vi "_old_Load_HW_globals.vi"(0 "HW settings path":path=path "C:/Experiment/Data Acquisition/Hardware Control/procedures/23Apr09_Example", 1 "Load pre 5.6 Globals?":bool, 2 "Pre 4.1 HWGlobals?":bool, 5 "error in":errorcluster) -> (6 "Loaded Procedure Data":T1={"User defined functions"="\n-- -------------------------------------------------------------------------------------------\n-- The following functions are part of the \"standard load\" of functions and should not be messed with\n-- They are here for reference only.\n-- Please add any user functions above this comment\n-- -------------------------------------------------------------------------------------------\n\n-- Creates a linear ramp from A to B\nfunction LineRamp(f, Initial, Final)\n    return (1-f)*Initial + f*Final;\nend\n\n-- Creates an exponential ramp from A to B\nfunction ExpRamp(t, a, b, tau)\n   return (b - a*exp(tMax / tau) + (a-b)*exp(t/tau))/ ( 1 - exp(tMax / tau) );\nend\n\n-- Creates a sinewave\nfunction SinRamp(t,Offset,A,Freq, Phase)\n    return Offset + A * sin(2*pi*Freq*t + Phase)\nend\n\n-- Creates a blackman pulse\nfunction Blackman(f, Offset, A)\n    return Offset +  A*sqrt(0.5*cos(3.1415*(2*f-1))+0.08*cos(2*pi*(2*f-1))+0.42);\nend\n\n-- Creates a half-gauss ramp\nfunction HalfGaussRamp(t, a, b, Width)\n    local y;\n    y = exp(-(tMax^2)/Width^2);\n    y = (a -  b*y)/(1-y)  +  ((b-a)/(1-y))*exp(-((t-tMax)^2)/Width^2);\n    return y;\nend\n\n-- Creates an \"O'Hara\" ramp from A to B, for dipole evaporation\nfunction EvapRamp(t, a, b, tau)\n   local y;\n  y = log(a/b) / log(1+tMax/tau);\n  y = a * (1+t/tau)^(-y);\n  return y;\nend\n", "Master AO Channels"=[], "Novatech Devices"=[], "DDS Devices"=[]}, 7 "Profile Name":string="IBS_PICameraTest_29Sep04", 8 "error out":errorcluster)   [LabVIEW 2013]
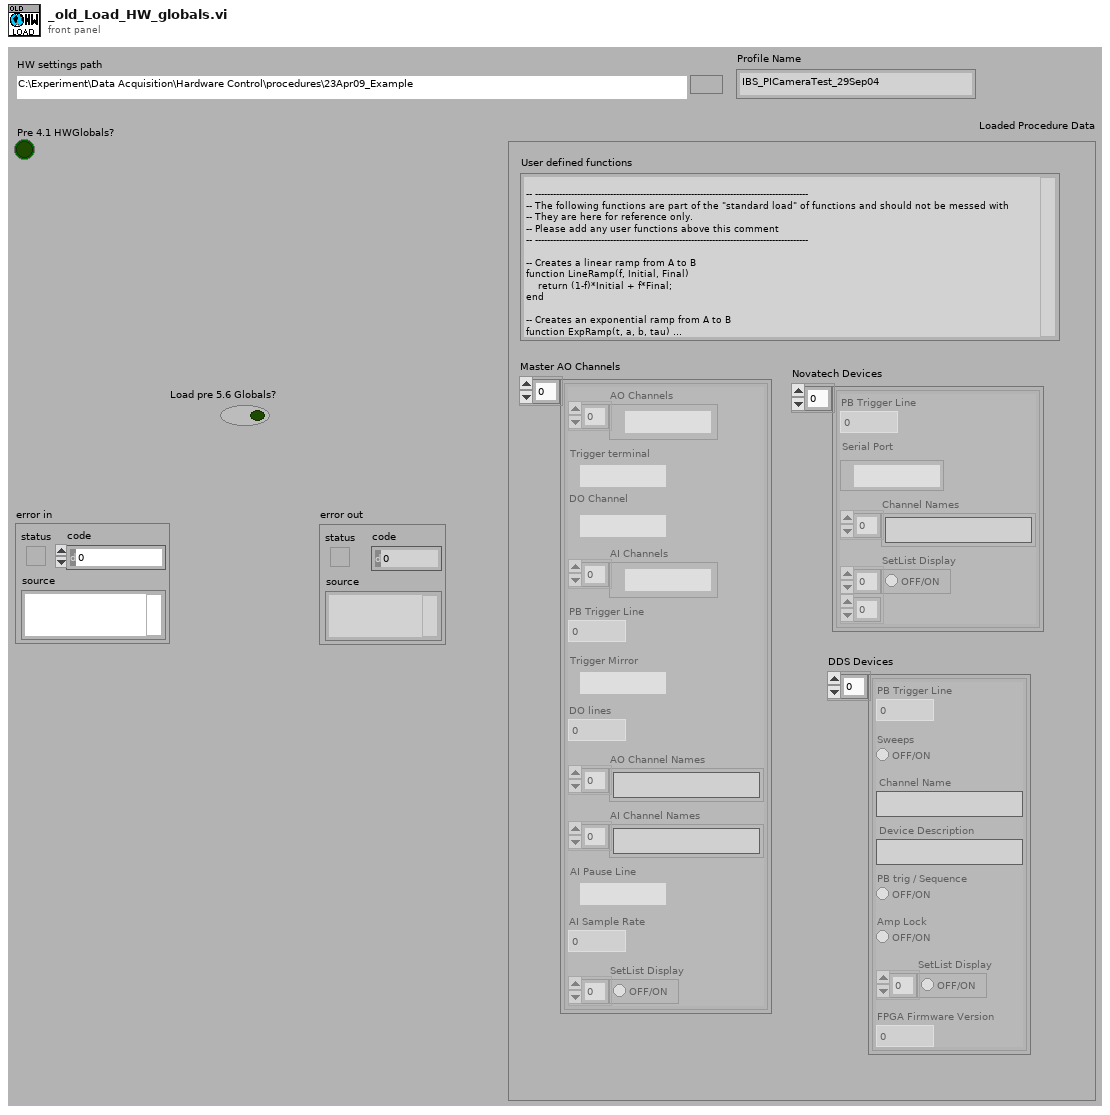
[diagram p1: front panel]
types:
  T1 = cluster{"User defined functions":string, "Master AO Channels":cluster{"AO Channels":refnum<k21>[], "Trigger terminal":tag, "DO Channel":refnum<k21>, "AI Channels":refnum<k21>[], "PB Trigger Line":u16, "Trigger Mirror":tag, "DO lines":i32, "AO Channel Names":string[], "AI Channel Names":string[], "AI Pause Line":tag, "AI Sample Rate":dbl, "SetList Display":bool[]}[], "Novatech Devices":cluster{"PB Trigger Line":u16, "Serial Port":refnum<visa-resource-name>, "Channel Names":string[], "SetList Display":bool[][]}[], "DDS Devices":cluster{"PB Trigger Line":u16, "Sweeps":bool, "Channel Name":string, "Device Description":string, "PB trig / Sequence":bool, "Amp Lock":bool, "SetList Display":bool[], "FPGA Firmware Version":dbl}[]}
  T2 = cluster{"PB Trigger Line":u16, "Serial Port":refnum<visa-resource-name>, "Channel Names":string[], "SetList Display":bool[][]}
  T3 = cluster{"AO Channels":refnum<k21>[], "Trigger terminal":tag, "DO Channel":refnum<k21>, "AI Channels":refnum<k21>[], "PB Trigger Line":u16, "Trigger Mirror":tag, "DO lines":i32, "AO Channel Names":string[], "AI Channel Names":string[], "AI Pause Line":tag, "AI Sample Rate":dbl, "SetList Display":bool[]}
  T4 = cluster{"PB Trigger Line":u16, "Sweeps":bool, "Channel Name":string, "Device Description":string, "PB trig / Sequence":bool, "Amp Lock":bool, "SetList Display":bool[], "FPGA Firmware Version":dbl}
  T5 = cluster{"PB Trigger Line":u16, "Sweeps":bool, "Channel Name":string, "Device Description":string, "PB trig / Sequence":bool, "Amp Lock":bool, "SetList Display":bool[], "FPGA Firmware Version":dbl}[]
  T6 = cluster{"PB Trigger Line":u16, "Sweeps":bool, "Channel Name":string, "Device Description":string, "PB trig / Sequence":bool, "Amp Lock":bool, "SetList Display":bool[]}
  T7 = cluster{"PB Trigger Line":u16, "Sweeps":bool, "Channel Name":string, "Device Description":string, "PB trig / Sequence":bool, "Amp Lock":bool, "SetList Display":bool[]}[]
  T8 = cluster{"PB Trigger Line":u16, "Serial Port":refnum<visa-resource-name>, "Channel Names":string[]}
  T9 = cluster{"PB Trigger Line":u16, "Serial Port":refnum<visa-resource-name>, "Channel Names":string[], "SetList Display":bool[][]}[]
  T10 = cluster{"AO Channels":refnum<k21>[], "Trigger terminal":tag, "DO Channel":refnum<k21>, "AI Channels":refnum<k21>[], "PB Trigger Line":u16, "Trigger Mirror":tag, "DO lines":i32, "AO Channel Names":string[], "AI Channel Names":string[], "AI Pause Line":tag, "AI Sample Rate":dbl}
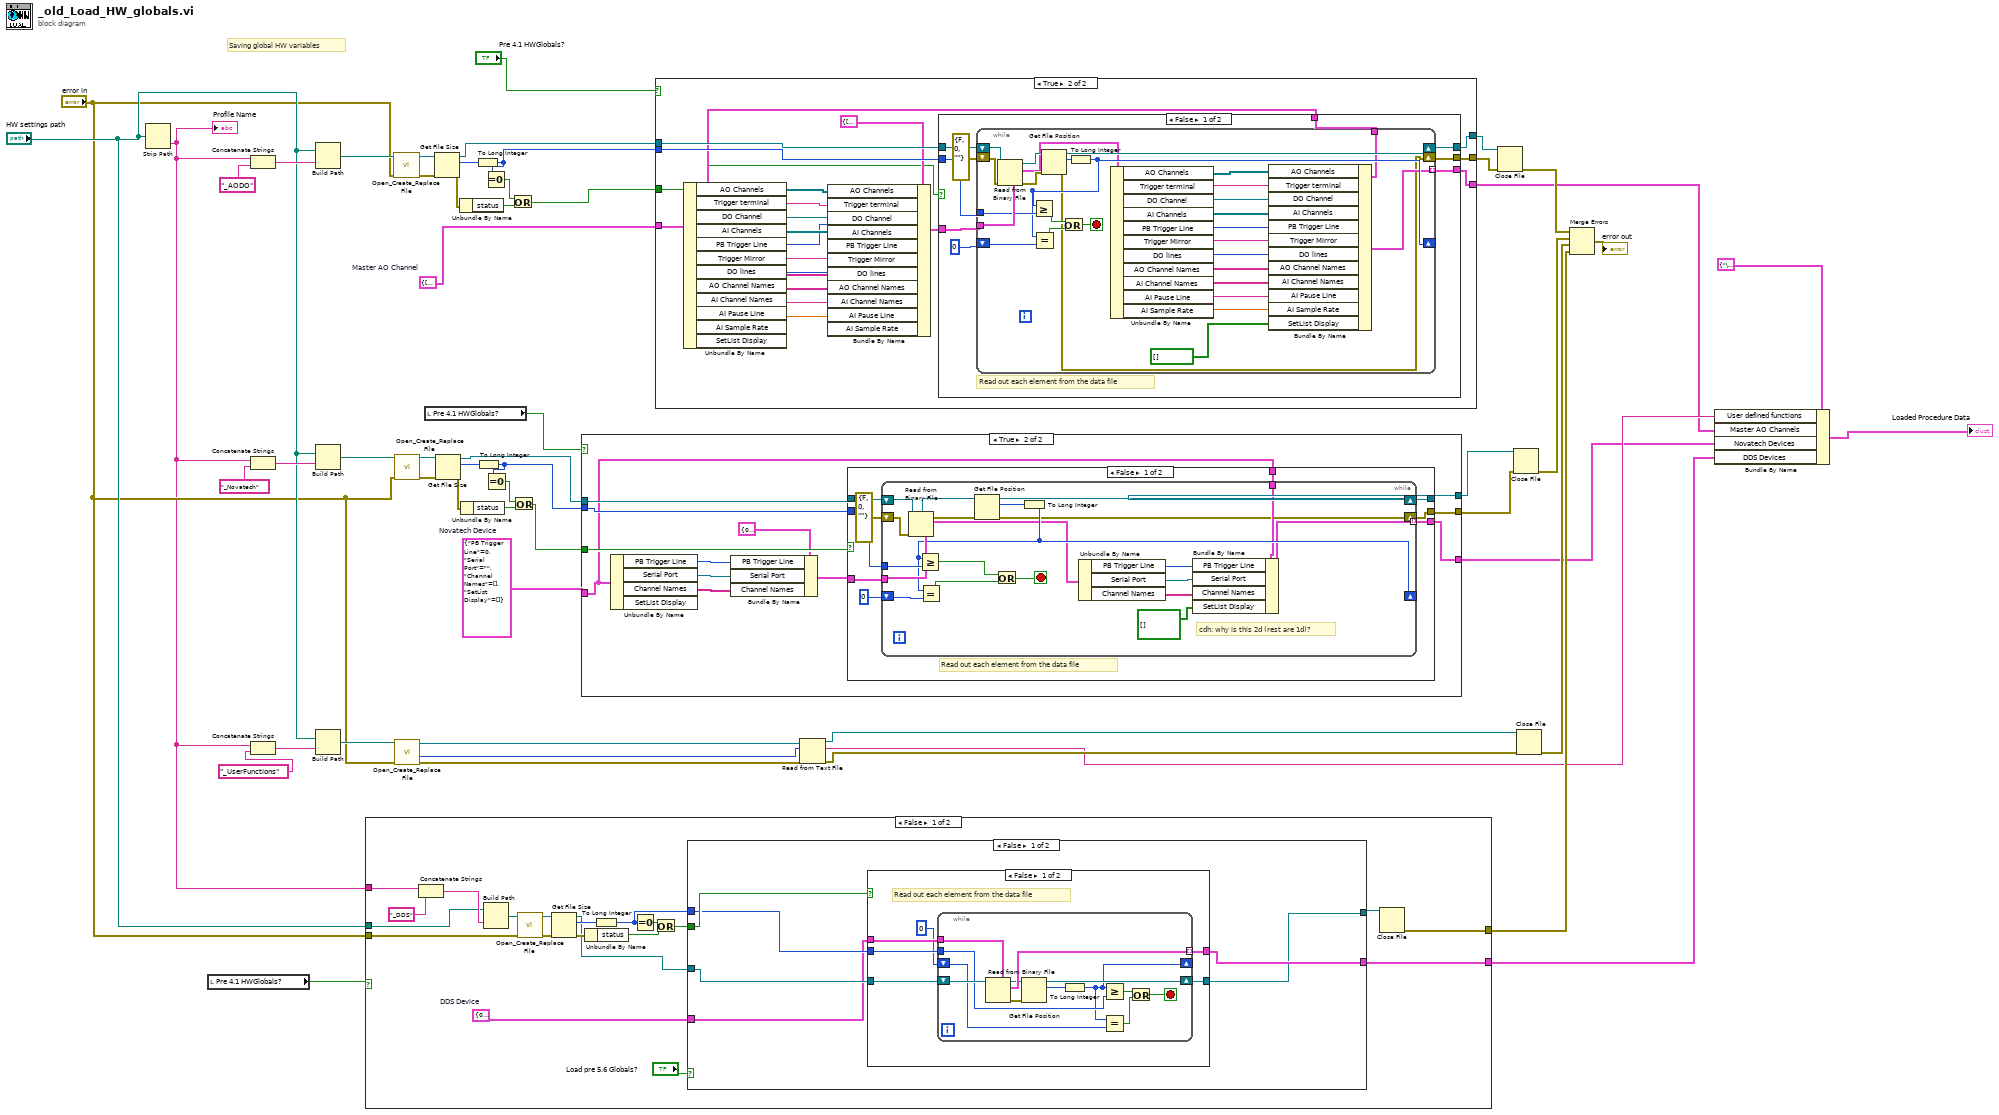
[diagram p0: block diagram]
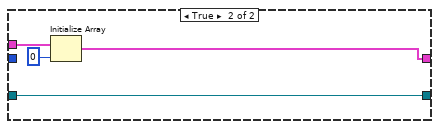
[diagram p2: hidden frame]
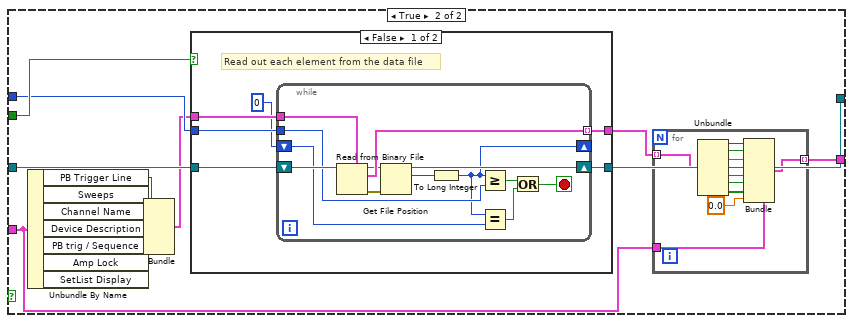
[diagram p3: hidden frame]
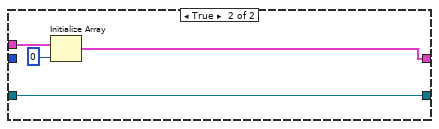
[diagram p4: hidden frame]
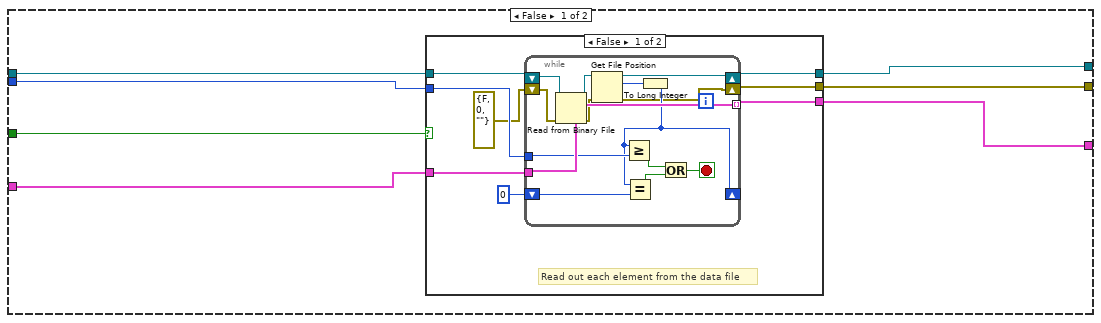
[diagram p6: hidden frame]
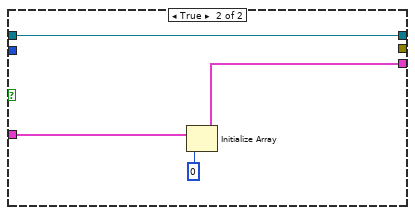
[diagram p7: hidden frame]
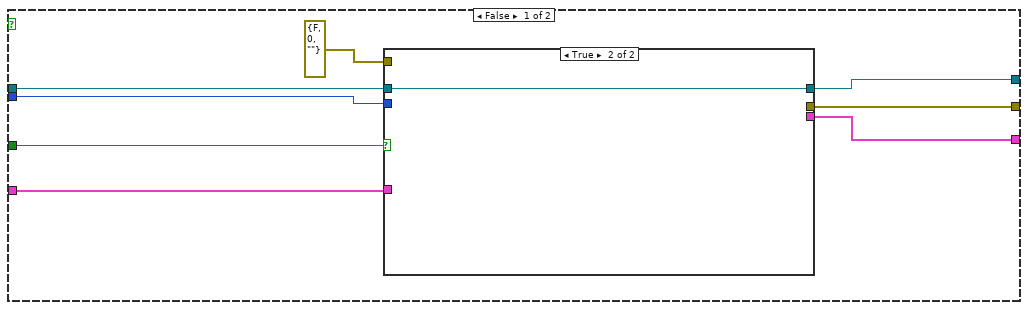
[diagram p9: hidden frame]
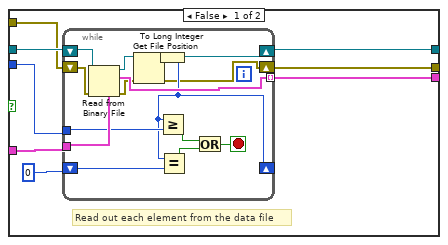
[diagram p10: hidden frame]
diagram:
  w5 = T2 {"PB Trigger Line"=0, "Serial Port"="", "Channel Names"=[], "SetList Display"=[]}  # Novatech Device
  w16 = T3 {"AO Channels"=[], "Trigger terminal"="", "DO Channel"="", "AI Channels"=[], "PB Trigger Line"=0, "Trigger Mirror"="", "DO lines"=0, "AO Channel Names"=[], "AI Channel Names"=[], "AI Pause Line"="", "AI Sample Rate"=0.0, "SetList Display"=[]}  # Master AO Channel
  # "Saving global HW variables"
  n1 = Strip Path(path="HW settings path") -> (name=w22:string)  [unwired: 1 out]
  "Profile Name" <- w22
  n2 = local read "Pre 4.1 HWGlobals?"() -> (w1:bool)
  n3 = Concatenate Strings(w22, "_AODO") -> (w54:string)
  n4 = Concatenate Strings(w22, "_Novatech") -> (w52:string)
  n5 = Concatenate Strings(w22, "_UserFunctions") -> (w33:string)
  n6 = Build Path(base path="HW settings path", name or relative path=w54) -> (appended path=w44:path)
  n7 = Build Path(base path="HW settings path", name or relative path=w52) -> (appended path=w37:path)
  n8 = Build Path(base path="HW settings path", name or relative path=w33) -> (appended path=w32:path)
  n9 = case shown="False" w1 {
    tunnel: "HW settings path" -> [w62 _]
    tunnel: "error in" -> [w61 _]
    tunnel: [w60 _] -> w23
    tunnel: w22 -> [w59 _]
    tunnel: [w56 _] -> w19
    frame False {
      w57 = T4 {"PB Trigger Line"=0, "Sweeps"=FALSE, "Channel Name"="", "Device Description"="", "PB trig / Sequence"=FALSE, "Amp Lock"=FALSE, "SetList Display"=[], "FPGA Firmware Version"=0.0}  # DDS Device
      n10 = Concatenate Strings(w59, "_DDS") -> (w64:string)
      n11 = Build Path(base path=w62, name or relative path=w64) -> (appended path=w75:path)
      n12 = call <vilib>:"Open_Create_Replace File.vi"("error in (no error)"=w61, "file path"=w75) -> ("error out"=w73:errorcluster, "refnum"=w66:refnum<file>)  [unwired: 4 in, 4 out]
      n13 = Get File Size(file=w66, error in=w73) -> (refnum out=w67:refnum<file>, size (in bytes)=w69:i64, 0:w74:errorcluster)
      n14 = Unbundle By Name(w74) -> ("status"=w72:bool)
      n15 = To Long Integer(number=w69) -> (32bit integer=w68:i32)
      n16 = Equal To 0?(x=w68) -> (x = 0?=w71:bool)
      n17 = Or(x=w71, y=w72) -> (x .or. y?=w70:bool)
      n18 = case shown="False" "Load pre 5.6 Globals?" {
        tunnel: w70 -> [w80 w119]
        tunnel: w68 -> [w79 w118]
        tunnel: w67 -> [w81 w117]
        tunnel: [w76 w116] -> w65
        tunnel: w57 -> [w78 w106]
        tunnel: [w77 w105] -> w56
        frame False {
          n19 = case shown="False" w80 {
            tunnel: [w87 w104] -> w76
            tunnel: w78 -> [w86 w102]
            tunnel: w81 -> [w85 w104]
            tunnel: [w84 w103] -> w77
            tunnel: w79 -> [w83 _]
            frame False {
              # "Read out each element from the data file"
              n20 = while {
                tunnel: [w98] -> w84 mode=indexing
                tunnel: w86 -> [w97]
                shift-right: [w99] -> w87
                shift-left: w85 -> [w100]
                tunnel: w83 -> [w96]
                shift-right: [w95] -> _
                shift-left: 0 -> [w94]
                stop <- w91 stop-if-true
                n21 = Read from Binary File(5:w97, 11:w100) -> (0:w89:errorcluster, 2:w98:T4, 3:w90:refnum<file>)  [unwired: 1 in, 4 out]
                n22 = Get File Position(4:w89, 7:w90) -> (2:w88:i64, 3:w99:refnum<file>)  [unwired: 1 out]
                n23 = To Long Integer(number=w88) -> (32bit integer=w95:i32)
                n24 = Greater Or Equal?(x=w95, y=w96) -> (x >= y?=w92:bool)
                n25 = Equal?(x=w95, y=w94) -> (x = y?=w93:bool)
                n26 = Or(x=w92, y=w93) -> (x .or. y?=w91:bool)
              }
            }
            frame True {
              n27 = Initialize Array(w102, 0) -> (w103:T5)
            }
          }
        }
        frame True {
          n28 = Unbundle By Name(w106) -> ("PB Trigger Line"=w109:u16, "Sweeps"=w115:bool, "Channel Name"=w114:string, "Device Description"=w113:string, "PB trig / Sequence"=w112:bool, "Amp Lock"=w111:bool, "SetList Display"=w110:bool[])
          n29 = Bundle("PB Trigger Line"=w109, "Sweeps"=w115, "Channel Name"=w114, "Device Description"=w113, "PB trig / Sequence"=w112, "Amp Lock"=w111, "SetList Display"=w110) -> (w108:T6)  [unwired: 1 in]
          n30 = case shown="False" w119 {
            tunnel: [w136 w153] -> w116
            tunnel: w108 -> [w135 w151]
            tunnel: w117 -> [w134 w153]
            tunnel: [w133 w152] -> w107
            tunnel: w118 -> [w132 _]
            frame False {
              # "Read out each element from the data file"
              n31 = while {
                tunnel: [w147] -> w133 mode=indexing
                tunnel: w135 -> [w146]
                shift-right: [w148] -> w136
                shift-left: w134 -> [w149]
                tunnel: w132 -> [w145]
                shift-right: [w144] -> _
                shift-left: 0 -> [w143]
                stop <- w140 stop-if-true
                n32 = Read from Binary File(5:w146, 11:w149) -> (0:w138:errorcluster, 2:w147:T6, 3:w139:refnum<file>)  [unwired: 1 in, 4 out]
                n33 = Get File Position(4:w138, 7:w139) -> (2:w137:i64, 3:w148:refnum<file>)  [unwired: 1 out]
                n34 = To Long Integer(number=w137) -> (32bit integer=w144:i32)
                n35 = Greater Or Equal?(x=w144, y=w145) -> (x >= y?=w141:bool)
                n36 = Equal?(x=w144, y=w143) -> (x = y?=w142:bool)
                n37 = Or(x=w141, y=w142) -> (x .or. y?=w140:bool)
              }
            }
            frame True {
              n38 = Initialize Array(w151, 0) -> (w152:T7)
            }
          }
          n39 = for {
            tunnel: w107 -> [w130] mode=indexing
            tunnel: w106 -> [w129]
            tunnel: [w120] -> w105 mode=indexing
            n40 = Unbundle(w130) -> ("PB Trigger Line"=w128:u16, "Sweeps"=w127:bool, "Channel Name"=w126:string, "Device Description"=w125:string, "PB trig / Sequence"=w124:bool, "Amp Lock"=w123:bool, "SetList Display"=w122:bool[])
            n41 = Bundle(cluster=w129, "PB Trigger Line"=w128, "Sweeps"=w127, "Channel Name"=w126, "Device Description"=w125, "PB trig / Sequence"=w124, "Amp Lock"=w123, "SetList Display"=w122, "FPGA Firmware Version"=0.0) -> (w120:T4)
          }
        }
      }
      n42 = Close File(refnum=w65) -> (error out=w60:errorcluster)  [unwired: 1 in, 1 out]
    }
    frame True {
    }
  }
  n43 = call <vilib>:"Open_Create_Replace File.vi"("error in (no error)"="error in", "file path"=w44) -> ("error out"=w46:errorcluster, "refnum"=w50:refnum<file>)  [unwired: 4 in, 4 out]
  n44 = call <vilib>:"Open_Create_Replace File.vi"("error in (no error)"="error in", "file path"=w37) -> ("error out"=w39:errorcluster, "refnum"=w43:refnum<file>)  [unwired: 4 in, 4 out]
  n45 = call <vilib>:"Open_Create_Replace File.vi"("error in (no error)"="error in", "file path"=w32) -> ("error out"=w28:errorcluster, "file size (bytes)"=w29:i32, "refnum"=w30:refnum<file>)  [unwired: 4 in, 3 out]
  n46 = local read "Pre 4.1 HWGlobals?"() -> (w6:bool)
  n47 = Get File Size(file=w50, error in=w46) -> (refnum out=w14:refnum<file>, size (in bytes)=w49:i64, 0:w45:errorcluster)
  n48 = Get File Size(file=w43, error in=w39) -> (refnum out=w7:refnum<file>, size (in bytes)=w42:i64, 0:w38:errorcluster)
  n49 = Unbundle By Name(w45) -> ("status"=w47:bool)
  n50 = Unbundle By Name(w38) -> ("status"=w40:bool)
  n51 = To Long Integer(number=w49) -> (32bit integer=w15:i32)
  n52 = To Long Integer(number=w42) -> (32bit integer=w8:i32)
  n53 = Equal To 0?(x=w15) -> (x = 0?=w48:bool)
  n54 = Equal To 0?(x=w8) -> (x = 0?=w41:bool)
  n55 = Or(x=w48, y=w47) -> (x .or. y?=w17:bool)
  n56 = Or(x=w41, y=w40) -> (x .or. y?=w9:bool)
  n57 = case shown="True" w6 {
    tunnel: [w160 w194] -> w2
    tunnel: w7 -> [w159 w195]
    tunnel: w8 -> [w158 w196]
    tunnel: w9 -> [w157 w193]
    tunnel: w5 -> [w156 w190]
    tunnel: [w155 w189] -> w4
    tunnel: [w154 w188] -> w3
    frame False {
      n58 = case shown="False" w157 {
        tunnel: [w168 w187] -> w160
        tunnel: w156 -> [w167 w185]
        tunnel: w159 -> [w166 w187]
        tunnel: [w165 w186] -> w155
        tunnel: w158 -> [w164 _]
        tunnel: [w162 _] -> w154
        frame False {
          # "Read out each element from the data file"
          n59 = while {
            tunnel: [w181] -> w165 mode=indexing
            tunnel: w167 -> [w180]
            shift-right: [w182] -> w168
            shift-left: w166 -> [w183]
            tunnel: w164 -> [w179]
            shift-right: [w178] -> _
            shift-left: 0 -> [w177]
            shift-right: [w170] -> w162
            shift-left: errorcluster {"status"=FALSE, "code"=0, "source"=""} ("error out") -> [w169]
            stop <- w174 stop-if-true
            n60 = Read from Binary File(5:w180, 8:w169, 11:w183) -> (0:w172:errorcluster, 2:w181:T2, 3:w173:refnum<file>)  [unwired: 4 out]
            n61 = Get File Position(4:w172, 7:w173) -> (0:w170:errorcluster, 2:w171:i64, 3:w182:refnum<file>)
            n62 = To Long Integer(number=w171) -> (32bit integer=w178:i32)
            n63 = Greater Or Equal?(x=w178, y=w179) -> (x >= y?=w175:bool)
            n64 = Equal?(x=w178, y=w177) -> (x = y?=w176:bool)
            n65 = Or(x=w175, y=w176) -> (x .or. y?=w174:bool)
          }
        }
        frame True {
          n66 = Initialize Array(w185, 0) -> (w186:T9)
        }
      }
    }
    frame True {
      n67 = Unbundle By Name(w190) -> ("PB Trigger Line"=w199:u16, "Serial Port"=w198:refnum<visa-resource-name>, "Channel Names"=w197:string[])  [unwired: 1 out]
      n68 = Bundle By Name(cluster=T8 {"PB Trigger Line"=0, "Serial Port"="", "Channel Names"=[]} ("output cluster"), "PB Trigger Line"=w199, "Serial Port"=w198, "Channel Names"=w197) -> (w191:T8)
      n69 = case shown="False" w193 {
        tunnel: [w208 w230] -> w194
        tunnel: w191 -> [w207 _]
        tunnel: w195 -> [w206 w230]
        tunnel: [w205 _] -> w189
        tunnel: w196 -> [w204 _]
        tunnel: w190 -> [w202 _]
        tunnel: [w201 _] -> w188
        frame False {
          # "Read out each element from the data file"
          n70 = while {
            tunnel: [w211] -> w205 mode=indexing
            tunnel: w207 -> [w227]
            shift-right: [w228] -> w208
            shift-left: w206 -> [w229]
            tunnel: w204 -> [w226]
            shift-right: [w225] -> _
            shift-left: 0 -> [w224]
            tunnel: w202 -> [w213]
            shift-right: [w210] -> w201
            shift-left: errorcluster {"status"=FALSE, "code"=0, "source"=""} ("error out") -> [w209]
            stop <- w221 stop-if-true
            # "cdh: why is this 2d (rest are 1d)?"
            n71 = Read from Binary File(5:w227, 8:w209, 11:w229) -> (0:w219:errorcluster, 2:w217:T8, 3:w220:refnum<file>)  [unwired: 4 out]
            n72 = Get File Position(4:w219, 7:w220) -> (0:w210:errorcluster, 2:w218:i64, 3:w228:refnum<file>)
            n73 = To Long Integer(number=w218) -> (32bit integer=w225:i32)
            n74 = Greater Or Equal?(x=w225, y=w226) -> (x >= y?=w222:bool)
            n75 = Equal?(x=w225, y=w224) -> (x = y?=w223:bool)
            n76 = Or(x=w222, y=w223) -> (x .or. y?=w221:bool)
            n77 = Unbundle By Name(w217) -> ("PB Trigger Line"=w216:u16, "Serial Port"=w215:refnum<visa-resource-name>, "Channel Names"=w214:string[])
            n78 = Bundle By Name(cluster=w213, "PB Trigger Line"=w216, "Serial Port"=w215, "Channel Names"=w214, "SetList Display"=bool[][] []) -> (w211:T2)
          }
        }
        frame True {
        }
      }
    }
  }
  n79 = case shown="True" "Pre 4.1 HWGlobals?" {
    tunnel: [w238 w280] -> w12
    tunnel: w14 -> [w237 w282]
    tunnel: w15 -> [w236 w281]
    tunnel: w17 -> [w235 w263]
    tunnel: w16 -> [w233 w265]
    tunnel: [w234 w266] -> w10
    tunnel: [w232 w264] -> w11
    frame False {
      n80 = case shown="True" w235 {
        tunnel: [w246 w262] -> w238
        tunnel: w233 -> [w245 _]
        tunnel: w237 -> [w244 w262]
        tunnel: [w243 _] -> w234
        tunnel: w236 -> [w242 _]
        tunnel: [w240 _] -> w232
        tunnel: errorcluster {"status"=FALSE, "code"=0, "source"=""} ("error out") -> [w239 _]
        frame False {
          # "Read out each element from the data file"
          n81 = while {
            tunnel: [w259] -> w243 mode=indexing
            tunnel: w245 -> [w258]
            shift-right: [w260] -> w246
            shift-left: w244 -> [w261]
            tunnel: w242 -> [w257]
            shift-right: [w256] -> _
            shift-left: 0 -> [w255]
            shift-right: [w248] -> w240
            shift-left: w239 -> [w247]
            stop <- w252 stop-if-true
            n82 = Read from Binary File(5:w258, 8:w247, 11:w261) -> (0:w250:errorcluster, 2:w259:T3, 3:w251:refnum<file>)  [unwired: 4 out]
            n83 = Get File Position(4:w250, 7:w251) -> (0:w248:errorcluster, 2:w249:i64, 3:w260:refnum<file>)
            n84 = To Long Integer(number=w249) -> (32bit integer=w256:i32)
            n85 = Greater Or Equal?(x=w256, y=w257) -> (x >= y?=w253:bool)
            n86 = Equal?(x=w256, y=w255) -> (x = y?=w254:bool)
            n87 = Or(x=w253, y=w254) -> (x .or. y?=w252:bool)
          }
        }
        frame True {
        }
      }
    }
    frame True {
      n88 = Unbundle By Name(w265) -> ("AO Channels"=w279:refnum<k21>[], "Trigger terminal"=w278:tag, "DO Channel"=w277:refnum<k21>, "AI Channels"=w276:refnum<k21>[], "PB Trigger Line"=w275:u16, "Trigger Mirror"=w274:tag, "DO lines"=w273:i32, "AO Channel Names"=w272:string[], "AI Channel Names"=w271:string[], "AI Pause Line"=w270:tag, "AI Sample Rate"=w269:dbl)  [unwired: 1 out]
      n89 = Bundle By Name(cluster=T10 {"AO Channels"=[], "Trigger terminal"="", "DO Channel"="", "AI Channels"=[], "PB Trigger Line"=0, "Trigger Mirror"="", "DO lines"=0, "AO Channel Names"=[], "AI Channel Names"=[], "AI Pause Line"="", "AI Sample Rate"=0.0} ("output cluster"), "AO Channels"=w279, "Trigger terminal"=w278, "DO Channel"=w277, "AI Channels"=w276, "PB Trigger Line"=w275, "Trigger Mirror"=w274, "DO lines"=w273, "AO Channel Names"=w272, "AI Channel Names"=w271, "AI Pause Line"=w270, "AI Sample Rate"=w269) -> (w268:T10)
      n90 = case shown="False" w263 {
        tunnel: [w291 w321] -> w280
        tunnel: w268 -> [w290 _]
        tunnel: w282 -> [w289 w321]
        tunnel: [w288 _] -> w266
        tunnel: w281 -> [w287 _]
        tunnel: w265 -> [w285 _]
        tunnel: [w284 _] -> w264
        frame False {
          # "Read out each element from the data file"
          n91 = while {
            tunnel: [w295] -> w288 mode=indexing
            tunnel: w290 -> [w318]
            shift-right: [w319] -> w291
            shift-left: w289 -> [w320]
            tunnel: w287 -> [w317]
            shift-right: [w316] -> _
            shift-left: 0 -> [w315]
            tunnel: w285 -> [w307]
            shift-right: [w293] -> w284
            shift-left: errorcluster {"status"=FALSE, "code"=0, "source"=""} ("error out") -> [w292]
            stop <- w312 stop-if-true
            n92 = Read from Binary File(5:w318, 8:w292, 11:w320) -> (0:w310:errorcluster, 2:w308:T10, 3:w311:refnum<file>)  [unwired: 4 out]
            n93 = Get File Position(4:w310, 7:w311) -> (0:w293:errorcluster, 2:w309:i64, 3:w319:refnum<file>)
            n94 = To Long Integer(number=w309) -> (32bit integer=w316:i32)
            n95 = Greater Or Equal?(x=w316, y=w317) -> (x >= y?=w313:bool)
            n96 = Equal?(x=w316, y=w315) -> (x = y?=w314:bool)
            n97 = Or(x=w313, y=w314) -> (x .or. y?=w312:bool)
            n98 = Unbundle By Name(w308) -> ("AO Channels"=w306:refnum<k21>[], "Trigger terminal"=w305:tag, "DO Channel"=w304:refnum<k21>, "AI Channels"=w303:refnum<k21>[], "PB Trigger Line"=w302:u16, "Trigger Mirror"=w301:tag, "DO lines"=w300:i32, "AO Channel Names"=w299:string[], "AI Channel Names"=w298:string[], "AI Pause Line"=w297:tag, "AI Sample Rate"=w296:dbl)
            n99 = Bundle By Name(cluster=w307, "AO Channels"=w306, "Trigger terminal"=w305, "DO Channel"=w304, "AI Channels"=w303, "PB Trigger Line"=w302, "Trigger Mirror"=w301, "DO lines"=w300, "AO Channel Names"=w299, "AI Channel Names"=w298, "AI Pause Line"=w297, "AI Sample Rate"=w296, "SetList Display"=bool[] []) -> (w295:T3)
          }
        }
        frame True {
        }
      }
    }
  }
  n100 = Read from Text File(file (use dialog)=w30, count=w29, error in=w28) -> (refnum out=w27:refnum<file>, text=w20:string, error out=w26:errorcluster)  [unwired: 2 out]
  n101 = Close File(refnum=w12, error in=w11) -> (error out=w35:errorcluster)  [unwired: 1 out]
  n102 = Close File(refnum=w2, error in=w3) -> (error out=w36:errorcluster)  [unwired: 1 out]
  n103 = Close File(refnum=w27, error in=w26) -> (error out=w31:errorcluster)  [unwired: 1 out]
  n104 = Merge Errors(w35, w36, w31, w23) -> (→"error out":errorcluster)
  n105 = Bundle By Name(cluster=T1 {"User defined functions"="\n-- -------------------------------------------------------------------------------------------\n-- The following functions are part of the \"standard load\" of functions and should not be messed with\n-- They are here for reference only.\n-- Please add any user functions above this comment\n-- -------------------------------------------------------------------------------------------\n\n-- Creates a linear ramp from A to B\nfunction LineRamp(f, Initial, Final)\n    return (1-f)*Initial + f*Final;\nend\n\n-- Creates an exponential ramp from A to B\nfunction ExpRamp(t, a, b, tau)\n   return (b - a*exp(tMax / tau) + (a-b)*exp(t/tau))/ ( 1 - exp(tMax / tau) );\nend\n\n-- Creates a sinewave\nfunction SinRamp(t,Offset,A,Freq, Phase)\n    return Offset + A * sin(2*pi*Freq*t + Phase)\nend\n\n-- Creates a blackman pulse\nfunction Blackman(f, Offset, A)\n    return Offset +  A*sqrt(0.5*cos(3.1415*(2*f-1))+0.08*cos(2*pi*(2*f-1))+0.42);\nend\n\n-- Creates a half-gauss ramp\nfunction HalfGaussRamp(t, a, b, Width)\n    local y;\n    y = exp(-(tMax^2)/Width^2);\n    y = (a -  b*y)/(1-y)  +  ((b-a)/(1-y))*exp(-((t-tMax)^2)/Width^2);\n    return y;\nend\n\n-- Creates an \"O'Hara\" ramp from A to B, for dipole evaporation\nfunction EvapRamp(t, a, b, tau)\n   local y;\n  y = log(a/b) / log(1+tMax/tau);\n  y = a * (1+t/tau)^(-y);\n  return y;\nend\n", "Master AO Channels"=[], "Novatech Devices"=[], "DDS Devices"=[]} ("Loaded Procedure Data"), "User defined functions"=w20, "Master AO Channels"=w10, "Novatech Devices"=w4, "DDS Devices"=w19) -> (→"Loaded Procedure Data":T1)
